vi "Tortoisegit Exists.vi"() -> (2 "file or folder exists?":bool, 3 "TortoiseGitProc.exe":path)   [LabVIEW 2017]
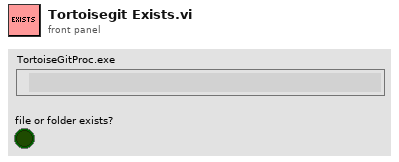
[diagram p1: front panel]
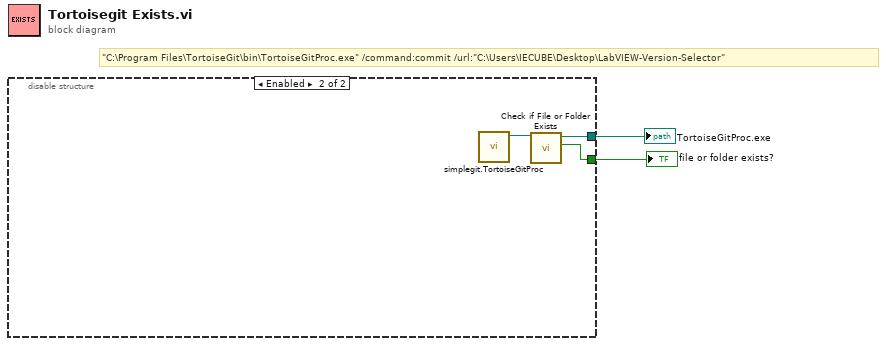
[diagram p0: block diagram]
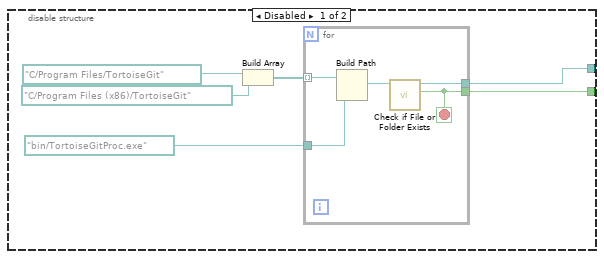
[diagram p2: hidden frame]
diagram:
  # "\"C:\\Program Files\\TortoiseGit\\bin\\TortoiseGitProc.exe\" /command:commit /url:\"C:\\Users\\IECUBE\\Desktop\\LabVIEW-Version-Selector\""
  n1 = disable-structure shown="Enabled" {
    disable-tunnel: [w4 w15] -> w2
    disable-tunnel: [w3 w16] -> w1
    frame Disabled {
      n2 = Build Array(path "C:/Program Files/TortoiseGit", path "C:/Program Files (x86)/TortoiseGit") -> (w6:path[])
      n3 = for {
        tunnel: w6 -> [w13] mode=indexing
        tunnel: path "bin/TortoiseGitProc.exe" -> [w12]
        tunnel: [w10] -> w3
        tunnel: [w9] -> w4
        stop <- w9 stop-if-true
        n4 = Build Path(base path=w13, name or relative path=w12) -> (appended path=w11:path)
        n5 = call <vilib>:"Check if File or Folder Exists.vi"("path"=w11) -> ("file or folder exists?"=w9:bool, "dup path"=w10:path)  [unwired: 8 in, 1 out]
      }
    }
    frame Enabled {
      n6 = call "simplegit.TortoiseGitProc.vi"() -> ("Path"=w14:path)  [unwired: 11 in]
      n7 = call <vilib>:"Check if File or Folder Exists.vi"("path"=w14) -> ("file or folder exists?"=w15:bool, "dup path"=w16:path)  [unwired: 8 in, 1 out]
    }
  }
  "file or folder exists?" <- w2
  "TortoiseGitProc.exe" <- w1
